vi "Clear Warning.vi"(8 "error in (no error)":errorcluster) -> (0 "cleared warning or error dup":errorcluster, 3 "error in (dup)":errorcluster)   [LabVIEW 2021, in "Error.lvlib"]
doc: "This VI output an \"no error\" cluster as <B>cleared warning or error dup</B> if the input cluster is a warning, otherwise it leaves the input error cluster untouched.\n\nThe <b>error in (dup)</B> cluster is a copy of the input cluster, and is therefore where the copy of the clearer warning can be found.\n\nUse this VI to clear a warning when the following node overreacts to warnings (such as the Python Node, which interprets this as an error)."
uses:
  Error.lvlib
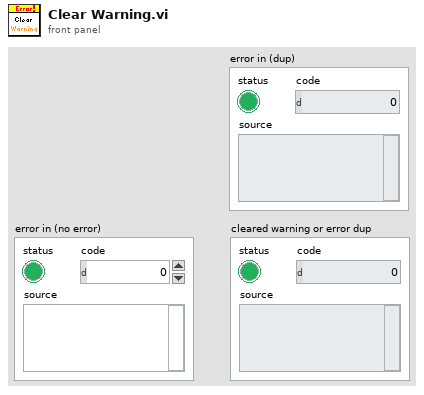
[diagram p1: front panel]
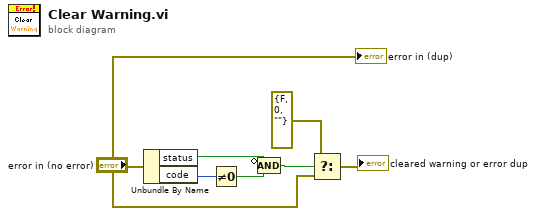
[diagram p0: block diagram]
diagram:
  n1 = Unbundle By Name("error in (no error)") -> ("status"=w5:bool, "code"=w7:i32)
  n2 = Not Equal To 0?(x=w7) -> (x != 0?=w6:bool)
  n3 = Compound Arithmetic op=AND(invert w5, w6) -> (w3:bool)
  n4 = Select(t=errorcluster {"status"=FALSE, "code"=0, "source"=""} ("error out"), s=w3, f="error in (no error)") -> (s? t:f=→"cleared warning or error dup":errorcluster)
  "error in (dup)" <- "error in (no error)"
